vi "HEWH Remove Zeros.vi"(8 "error in (no error)":errorcluster, 10 "Index":i32, 11 "RTD Out Full Data\nSet (Each Draw)":dbl[][](array[numeric])) -> (0 "error out":errorcluster, 3 "Output":dbl[](array[numeric]))   [LabVIEW 2023]
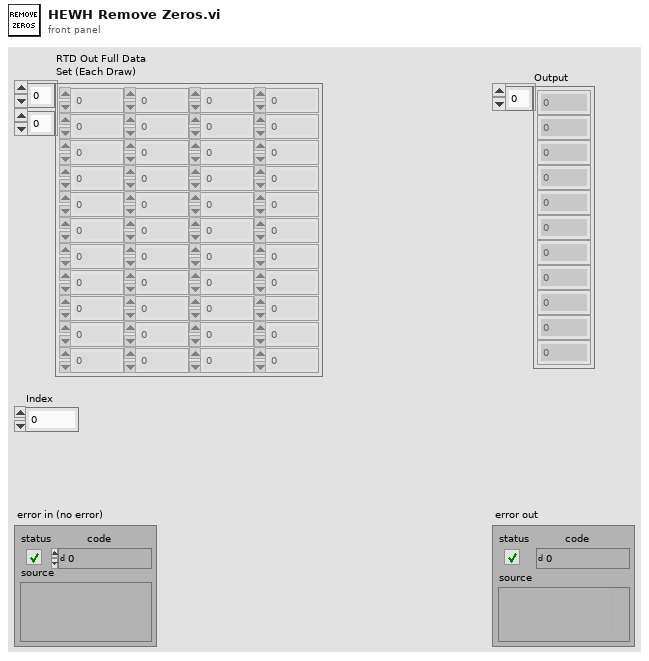
[diagram p1: front panel]
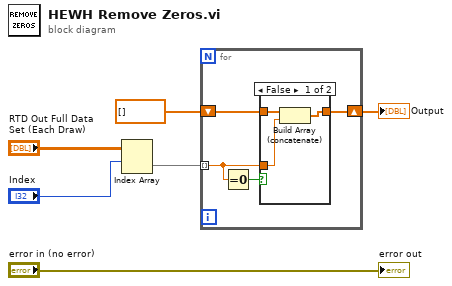
[diagram p0: block diagram]
diagram:
  n1 = Index Array "Index Array"(array="RTD Out Full Data\nSet (Each Draw)", index (row)="Index") -> (element=w3:dbl[])  [unwired: 1 in]
  n2 = for {
    tunnel: w3 -> [w7] mode=indexing
    shift-right: [w8] -> w5
    shift-left: dbl[] [] -> [w9]
    n3 = Equal To 0?(x=w7) -> (x = 0?=w10:bool)
    n4 = case shown="False" w10 {
      tunnel: w9 -> [w13 w14]
      tunnel: [w12 w14] -> w8
      tunnel: w7 -> [w11 _]
      frame False {
        n5 = Build Array (concatenate)(w13, w11) -> (w12:dbl[])
      }
      frame True {
      }
    }
  }
  "Output" <- w5
  "error out" <- "error in (no error)"
